vi "Init Muxes.vi"(8 "error in (no error)":errorcluster, 11 "MuxActor in":refnum<class "MuxActor.lvclass">) -> (0 "error out":errorcluster, 3 "MuxActor out":refnum<class "MuxActor.lvclass">)   [LabVIEW 2022 SP3, in "VideoMux.lvlib" / "MuxActor.lvclass"]
uses:
  MuxActor.lvclass
  <vilib>/IlluminatedG/IG Serial Stream/Stream-Serial/Serial Client/Port Config.ctl
  <vilib>/IlluminatedG/IG Serial Stream/Stream-Serial/Serial Client/Stop Bits.ctl
  <vilib>/IlluminatedG/IG Serial Stream/Stream-Serial/Serial Client/Flow Control.ctl
  <vilib>/IlluminatedG/IG Serial Stream/Stream-Serial/Serial Client/Parity.ctl
  <vilib>/Instr/_visa.llb/VISA Find Search Mode.ctl
  MuxActor.lvclass/MuxActor.ctl
  <vilib>/IlluminatedG/IG Serial Stream/Stream-Serial/Serial Client/Serial Client.lvclass
  C:/Program Files (x86)/National Instruments/LabVIEW 2022/vi.lib/IlluminatedG/lv-stream/Connection/Connection.lvclass
  Mux/Mux.lvclass
  <vilib>/IlluminatedG/lv-stream/Connection/Connection.lvclass
  C:/Program Files (x86)/National Instruments/LabVIEW 2022/vi.lib/IlluminatedG/lv-stream/Endpoint/Endpoint.lvclass
  C:/Program Files (x86)/National Instruments/LabVIEW 2022/vi.lib/IlluminatedG/IG Serial Stream/Stream-Serial/Serial Client/Serial Client.lvclass
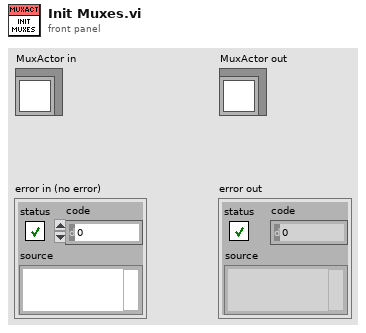
[diagram p1: front panel]
types:
  T1 = typedef "VISA Find Search Mode.ctl" = u32
  T2 = typedef "Stream-Serial.lvlib/Serial Client.lvclass/Port Config.ctl" = cluster{"Baud (115200)":u32, "Data Bits (8)":u8, "Stop Bits (1)":T3, "Flow Control":T4, "Use LineTerm?":bool, "LineTerm (\\n)":string, "Timeout ms (10000)":i32, "Parity (None)":T5}
  T3 = typedef "Stream-Serial.lvlib/Serial Client.lvclass/Stop Bits.ctl" = u16
  T4 = typedef "Stream-Serial.lvlib/Serial Client.lvclass/Flow Control.ctl" = u16
  T5 = typedef "Stream-Serial.lvlib/Serial Client.lvclass/Parity.ctl" = enum16{"None", "Odd", "Even", "Mark", "Space"}
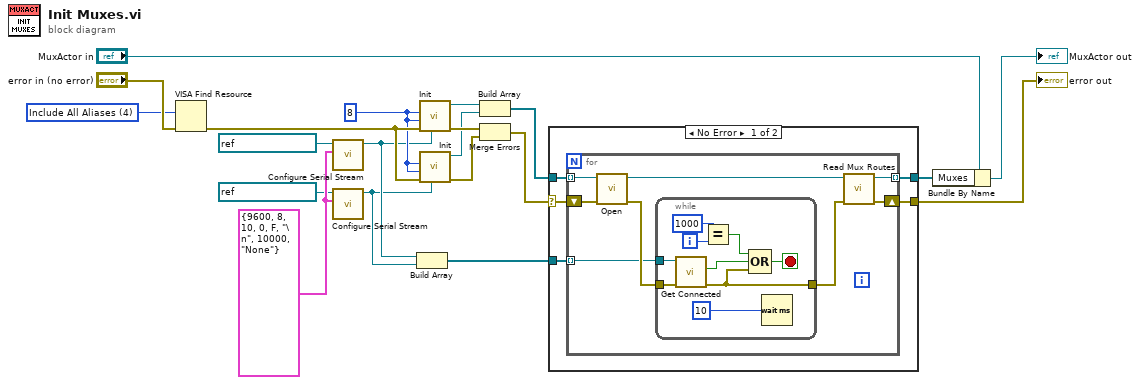
[diagram p0: block diagram]
diagram:
  w4 = T1 4 items=["Canonical Names Only"=0, "Aliases Only"=2, "Include Matching Aliases"=3, "Include All Aliases"=4] ("Search Mode")
  w15 = 8 ("In Count")
  w18 = T2 {"Baud (115200)"=9600, "Data Bits (8)"=8, "Stop Bits (1)"=10, "Flow Control"=0, "Use LineTerm?"=FALSE, "LineTerm (\\n)"="\n", "Timeout ms (10000)"=10000, "Parity (None)"=enum."None"} ("Port Config (115200 8N1)")
  n1 = VISA Find Resource(8:"error in (no error)", 10:w4) -> (0:w19:errorcluster)  [unwired: 1 in, 2 out]
  n2 = call <vilib>:"Configure Serial Stream.vi"("Port Config (115200 8N1)"=w18, "Serial Port"=refnum<visa-resource-name> "ASRL3::INSTR") -> ("Serial Client out"=w8:refnum<class "Serial Client.lvclass">)  [unwired: 8 in, 1 out]
  n3 = call <vilib>:"Configure Serial Stream.vi"("Port Config (115200 8N1)"=w18, "Serial Port"=refnum<visa-resource-name> "ASRL4::INSTR") -> ("Serial Client out"=w7:refnum<class "Serial Client.lvclass">)  [unwired: 8 in, 1 out]
  n4 = Build Array(w8, w7) -> (w6:refnum<class "Serial Client.lvclass">[])
  n5 = call "Init.vi"("Connection"=w8, "error in (no error)"=w19, "Out Count"=w15, "In Count"=w15) -> ("error out"=w14:errorcluster, "Mux out"=w12:refnum<class "Mux.lvclass">)  [unwired: 6 in]
  n6 = call "Init.vi"("Connection"=w7, "error in (no error)"=w19, "Out Count"=w15, "In Count"=w15) -> ("error out"=w13:errorcluster, "Mux out"=w11:refnum<class "Mux.lvclass">)  [unwired: 6 in]
  n7 = Build Array(w12, w11) -> (w9:refnum<class "Mux.lvclass">[])
  n8 = Merge Errors(w14, w13) -> (w10:errorcluster)
  n9 = case shown="No Error" w10 {
    selector: w10 -> [w25 w44]
    tunnel: w9 -> [w24 w43]
    tunnel: [w23 w44] -> w1
    tunnel: w6 -> [w22 _]
    tunnel: [w21 w43] -> w5
    frame No Error {
      n10 = for {
        shift-right: [w27] -> w23
        shift-left: w25 -> [w32]
        tunnel: w24 -> [w31] mode=indexing
        tunnel: w22 -> [w30] mode=indexing
        tunnel: [w26] -> w21 mode=indexing
        n11 = call-dynamic "Open.vi"("error in (no error)"=w32, "Mux in"=w31) -> ("error out"=w33:errorcluster, "Mux out"=w29:refnum<class "Mux.lvclass">)  [unwired: 8 in]
        n12 = while {
          tunnel: w30 -> [w42]
          tunnel: [w37] -> w28
          tunnel: w33 -> [w39]
          i -> [w36]
          stop <- w38 stop-if-true
          n13 = call <vilib>:"Get Connected.vi"("error in (no error)"=w39, "Connection in"=w42) -> ("error out"=w37:errorcluster, "Connected"=w40:bool)  [unwired: 7 in, 1 out]
          n14 = Equal?(x=1000, y=w36) -> (x = y?=w34:bool)
          n15 = Compound Arithmetic op=OR(w34, w40, w37) -> (w38:bool)
          n16 = Wait (ms)(milliseconds to wait=u32 10) -> ()  [unwired: 1 out]
        }
        n17 = call-dynamic "Read Mux Routes.vi"("error in (no error)"=w28, "Mux in"=w29) -> ("error out"=w27:errorcluster, "Mux out"=w26:refnum<class "Mux.lvclass">)  [unwired: 7 in, 1 out]
      }
    }
    frame Error {
    }
  }
  "error out" <- w1
  n18 = Bundle By Name(cluster="MuxActor in", "Muxes"=w5) -> (→"MuxActor out":refnum<class "MuxActor.lvclass">)
